vi "convert type defs to channels.vi"(11 "fixed channel configuration":refnum<class "fixed channel configuration.lvclass">) -> (0 "error out":errorcluster, 3 "Array out":refnum<class "TBM channel.lvclass">[](array[class]))   [LabVIEW 2013, in "fixed channel configuration.lvclass"]
uses:
  fixed channel configuration.lvclass
  <vilib>/NI/Tag Bus Module Framework/channel/TBM channel.lvclass
  <vilib>/regexp/Match Regular Expression.xnode
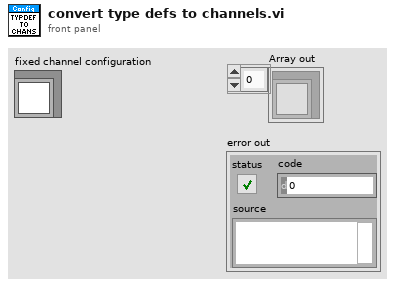
[diagram p1: front panel]
types:
  T1 = typedef "TBM channel.lvclass/channel classification.ctl" = enum16{"input data", "output data", "processing parameter", "processing result"}
  T2 = typedef "tag bus.lvlib/tag descriptor.lvclass/Data Type.ctl" = enum16{"Double", "Single", "I64", "I32", "I16", "I8", "U64", "U32", "U16", "U8", "Boolean", "String", "Array of Double", "Array of Single", "Array of I64", "Array of I32", "Array of I16", "Array of I8", "Array of U64", "Array of U32", "Array of U16", "Array of U8", "Array of Boolean", "Array of String"}
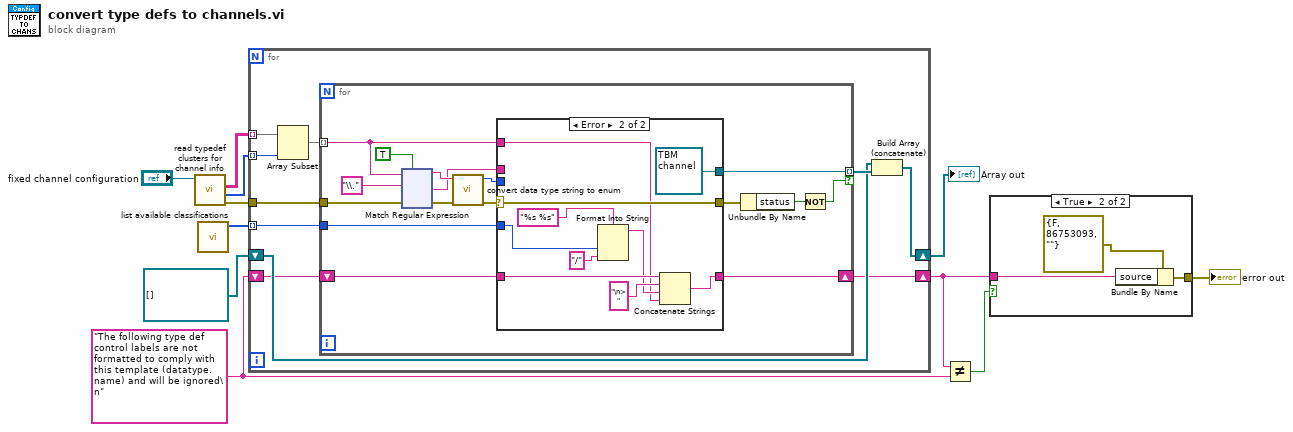
[diagram p0: block diagram]
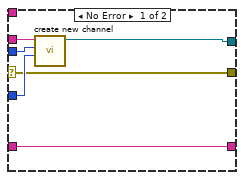
[diagram p3: hidden frame]
diagram:
  w8 = "The following type def control labels are not formatted to comply with this template (datatype.name) and will be ignored\n"
  n1 = call "read typedef clusters for channel info.vi"("fixed channel configuration"="fixed channel configuration") -> ("error out"=w6:errorcluster, "Channel Counts"=w3:i32[], "> Categorized name list >"=w5:string[][])  [unwired: 7 in, 1 out]
  n2 = call <vilib>:"list available classifications.vi"() -> ("supported types"=w1:T1[])  [unwired: 11 in]
  n3 = for {
    tunnel: w1 -> [w21] mode=indexing
    shift-right: [w19] -> w7
    shift-left: refnum<class "TBM channel.lvclass">[] [] -> [w18]
    tunnel: w5 -> [w14] mode=indexing
    tunnel: w6 -> [w17]
    shift-right: [w15] -> w10
    shift-left: w8 -> [w16]
    tunnel: w3 -> [w13] mode=indexing
    n4 = Array Subset(array=w14, length=w13) -> (w12:string[])  [unwired: 1 in]
    n5 = for {
      tunnel: w21 -> [w36]
      tunnel: [w37] -> w20 mode=indexing if=w27
      tunnel: w12 -> [w24] mode=indexing
      shift-right: [w22] -> w15
      shift-left: w16 -> [w23]
      tunnel: w17 -> [w33]
      n6 = xnode "Match Regular Expression"("input string"=w24, "regular expression"="\\.", "error in"=w33, "ignore case? (F)"=TRUE) -> ("before match"=w31:string, "after match"=w30:string, "error out"=w32:errorcluster)  [unwired: 2 in, 2 out]
      n7 = call "convert data type string to enum.vi"("error in"=w32, "Data Type String"=w31) -> ("error out"=w29:errorcluster, "Data Type Enum"=w25:T2)  [unwired: 8 in]
      n8 = case shown="Error" w29 {
        selector: w29 -> [w155 w166]
        tunnel: w36 -> [w157 w162]
        tunnel: [w155 w166] -> w28
        tunnel: [w156 refnum<class "TBM channel.lvclass"> refnum ("channel")] -> w37
        tunnel: w30 -> [w154 _]
        tunnel: w25 -> [w153 _]
        tunnel: w24 -> [_ w158]
        tunnel: w23 -> [w152 w165]
        tunnel: [w152 w164] -> w22
        frame No Error {
          n9 = call <vilib>:"create new channel.vi"("channel classification"=w157, "data type"=w153, "channel name"=w154) -> ("channel"=w156:refnum<class "TBM channel.lvclass">)  [unwired: 8 in]
        }
        frame Error {
          n10 = Format Into String(format string="%s %s", w162, "/") -> (resulting string=w159:string)  [unwired: 2 in, 1 out]
          n11 = Concatenate Strings(w165, "\n> " ("string"), w159, w158) -> (w164:string)
        }
      }
      n12 = Unbundle By Name(w28) -> ("status"=w26:bool)
      n13 = Not(x=w26) -> (.not. x?=w27:bool)
    }
    n14 = Build Array (concatenate)(w18, w20) -> (w19:refnum<class "TBM channel.lvclass">[])
  }
  "Array out" <- w7
  n15 = Not Equal?(x=w10, y=w8) -> (x != y?=w9:bool)
  n16 = case shown="True" w9 {
    tunnel: w10 -> [_ w169]
    tunnel: [_ w168] -> w11
    frame False {
    }
    frame True {
      n17 = Bundle By Name(cluster=errorcluster {"status"=FALSE, "code"=86753093, "source"=""} ("error constant"), "source"=w169) -> (w168:errorcluster)
    }
  }
  "error out" <- w11
